vi "Get Network Information.vi"(8 "error in (no error)":errorcluster, 11 "OK":bool) -> (0 "error out":errorcluster, 2 "Port number  out":u16=3363, 3 "Machine name out":string="localhost")   [LabVIEW 2013]
panel:
  in  "Cancel":bool
  in  "Machine name/IP":string="localhost"
  in  "Port number":u16=3363
  # "Enter Connection Information"
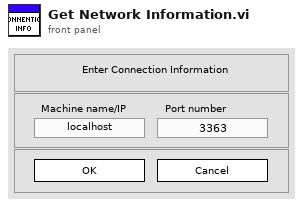
[diagram p1: front panel]
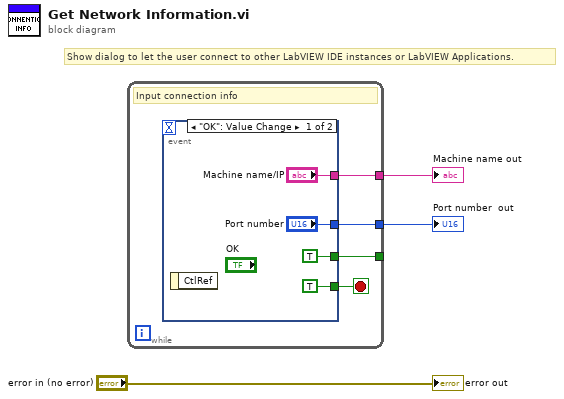
[diagram p0: block diagram]
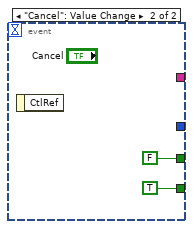
[diagram p2: hidden frame]
diagram:
  # "Show dialog to let the user connect to other LabVIEW IDE instances or LabVIEW Applications."
  n1 = while {
    tunnel: [w7] -> w2
    tunnel: [w6] -> w3
    tunnel: [w4] -> _
    stop <- w5 stop-if-true
    # "Input connection info"
    n2 = event shown="[0] \"OK\": Value Change" {
      selector: _ -> [_ _]
      dyn-events: _ -> [_ _]
      timeout: _ -> [_ _]
      tunnel: ["Port number" _] -> w7
      tunnel: ["Machine name/IP" _] -> w6
      tunnel: [TRUE TRUE] -> w5
      tunnel: [TRUE FALSE] -> w4
      event "OK": Value Change {
        n3 = event-data() -> ()  [unwired: 1 in, 1 out]
      }
      event "Cancel": Value Change {
        n4 = event-data() -> ()  [unwired: 1 in, 1 out]
      }
    }
  }
  "Port number  out" <- w2
  "Machine name out" <- w3
  "error out" <- "error in (no error)"
